vi "LanchAngleAndSpeed_with DRAG.vi"(3 "delta height (basket center-ball center) [m]":dbl, 4 "distance to center of basket (x axies)":dbl) -> (0 "initial velocity":dbl, 1 "pitching angle":dbl)   [LabVIEW 2011]
uses:
  <vilib>/express/express arith-compare/Formula/XNode/ExpressFormulaBlockNode.xnode
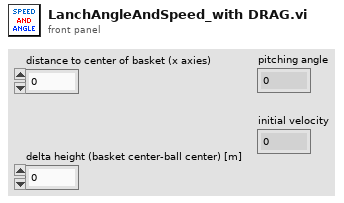
[diagram p1: front panel]
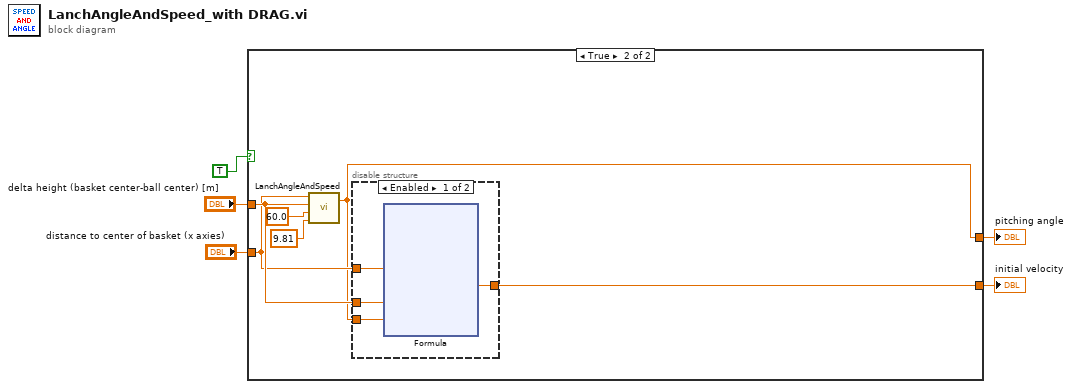
[diagram p0: block diagram]
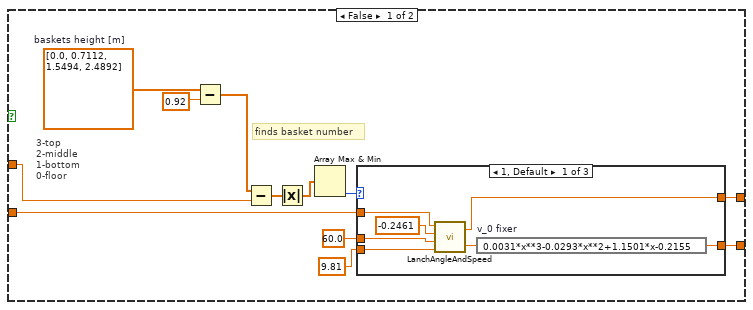
[diagram p2: hidden frame]
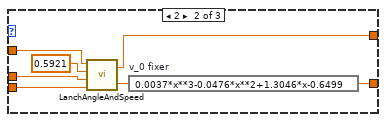
[diagram p3: hidden frame]
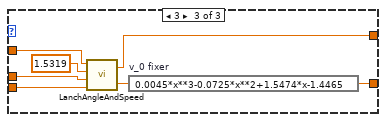
[diagram p4: hidden frame]
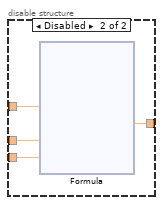
[diagram p5: hidden frame]
diagram:
  n1 = case shown="True" TRUE ("technique (T-new, F-old)") {
    tunnel: "distance to center of basket (x axies)" -> [w17 w41]
    tunnel: [w14 w39] -> w4
    tunnel: [w13 w40] -> w3
    tunnel: "delta height (basket center-ball center) [m]" -> [w10 w44]
    frame False {
      w7 = dbl[] [0.0, 0.7112, 1.5494, 2.4892]  # baskets height [m]
      # "finds basket number"
      # "3-top\n2-middle\n1-bottom\n0-floor"
      n2 = Subtract(x=w7, y=0.92) -> (x-y=w9:dbl[])
      n3 = Subtract(x=w9, y=w10) -> (x-y=w11:dbl[])
      n4 = Absolute Value(x=w11) -> (abs(x)=w12:dbl[])
      n5 = Array Max & Min(array=w12) -> (min index (indices)=w6:i32)  [unwired: 3 out]
      n6 = case shown="1, Default" w6 {
        tunnel: w17 -> [w23 w30 w37]
        tunnel: 60.0 ("b") -> [w22 w28 w35]
        tunnel: 9.81 ("g") -> [w21 w27 w34]
        tunnel: [w20 w26 w33] -> w14
        tunnel: [w18 w25 w32] -> w13
        frame 1, Default {
          n7 = call "LanchAngleAndSpeed.vi"("g"=w21, "entry angle"=w22, "height"=-0.2461, "horizontal distance"=w23) -> ("speed"=w19:dbl, "angle"=w20:dbl)
          n8 = expression code="0.0031*x**3-0.0293*x**2+1.1501*x-0.2155" "v_0 fixer"(w19) -> (w18:dbl)
        }
        frame 2 {
          n9 = call "LanchAngleAndSpeed.vi"("g"=w27, "entry angle"=w28, "height"=0.5921, "horizontal distance"=w30) -> ("speed"=w31:dbl, "angle"=w26:dbl)
          n10 = expression code="0.0037*x**3-0.0476*x**2+1.3046*x-0.6499" "v_0 fixer"(w31) -> (w25:dbl)
        }
        frame 3 {
          n11 = call "LanchAngleAndSpeed.vi"("g"=w34, "entry angle"=w35, "height"=1.5319, "horizontal distance"=w37) -> ("speed"=w38:dbl, "angle"=w33:dbl)
          n12 = expression code="0.0045*x**3-0.0725*x**2+1.5474*x-1.4465" "v_0 fixer"(w38) -> (w32:dbl)
        }
      }
    }
    frame True {
      n13 = call "LanchAngleAndSpeed.vi"("g"=9.81, "entry angle"=60.0 ("b"), "height"=w44, "horizontal distance"=w41) -> ("angle"=w39:dbl)  [unwired: 1 out]
      n14 = disable-structure shown="Enabled" {
        disable-tunnel: w44 -> [w48 w63]
        disable-tunnel: w41 -> [w47 w64]
        disable-tunnel: [w46 w61] -> w40
        disable-tunnel: w39 -> [w45 w62]
        frame Enabled {
          n15 = xnode "Formula"("R"=w47, "H"=w48, "a"=w45) -> ("Result"=w46:dbl)  [unwired: 1 in, 1 out]
        }
        frame Disabled {
          n16 = xnode "Formula"("R"=w64, "H"=w63, "a"=w62) -> ("Result"=w61:dbl)  [unwired: 1 in, 1 out]
        }
      }
    }
  }
  "pitching angle" <- w4
  "initial velocity" <- w3
